vi "Abstract MVA Application (Template).vi"   [LabVIEW 2015]
uses:
  Framework/IModel/IModel/IModel.lvclass
  Framework/IViewable/IViewable/IViewable.lvclass
  Framework/IViewModel/IViewModel/IViewModel.lvclass
  Framework/Mediator/Mediator/Mediator.lvclass
  Framework/Mediator/MediatorBusMonitor/MediatorBusMonitor.lvclass
  <vilib>/ActorFramework/Message Enqueuer/Message Priority.ctl
  Framework/IViewable/IViewable/View Position Enum.ctl
  Framework/IMediator/IMediator/IMediator.lvclass/IMediator.ctl
  Framework/IViewModel/IViewModel/IViewModel.lvclass/IViewModel.ctl
  Framework/IViewManager/IViewManager Messages/Launch Nested Views Msg/Launch Nested Views Msg.lvclass/Launch Nested Views Msg.ctl
  Framework/IViewManager/IViewManager/IViewManager.lvclass/IViewManager.ctl
  Framework/IViewable/IViewable Messages/Open Front Panel Msg/Open Front Panel Msg.lvclass/Open Front Panel Msg.ctl
  <vilib>/ActorFramework/Message Enqueuer/Message Enqueuer.lvclass/Message Enqueuer.ctl
  Framework/IViewManager/IViewManager Messages/Launch Nested Views Msg/Pack Launch Nested Views Msg.vi
  Framework/IViewManager/IViewManager/Write Startup Launch Nested Views Msg.vi
  <vilib>/ActorFramework/Message Enqueuer/Enqueue.vi
  <vilib>/ActorFramework/Message Priority Queue/Priority Enqueue.vi
  Framework/IViewable/IApplicationStyle/IApplicationStyle.lvclass
  Framework/IViewManager/IViewManager Messages/Launch Nested Views Msg/Launch Nested Views Msg.lvclass
  Framework/IViewable/IViewable Messages/Open Front Panel Msg/Open Front Panel Msg.lvclass
  <vilib>/ActorFramework/Actor/Actor.lvclass
  Framework/IMediator/IMediator/IMediator.lvclass
  <vilib>/ActorFramework/Message Enqueuer/Message Enqueuer.lvclass
panel:
  # "This example launches a simple abstract MVA application.\nReplace IModel with your Root Model or dependency-injected Model hierarchy.\nReplace IViewable with your Viewable or nested hierarchy of Viewables and ViewManagers\nReplace IViewModel with your concrete ViewModel that requests Model activity driven by user inputs\nMediator is already concrete--only replace it if you write your own Mediator (highly unlikely)"
types:
  T1 = typedef "IViewable.lvlib/IViewable.lvclass/View Position Enum.ctl" = enum16{"Centered", "Maximized", "Minimized", "Custom", "Unchanged"}
  T2 = typedef "Actor Framework.lvlib/Message Enqueuer.lvclass/Message Priority.ctl" = enum16{"Low", "Normal", "High"}
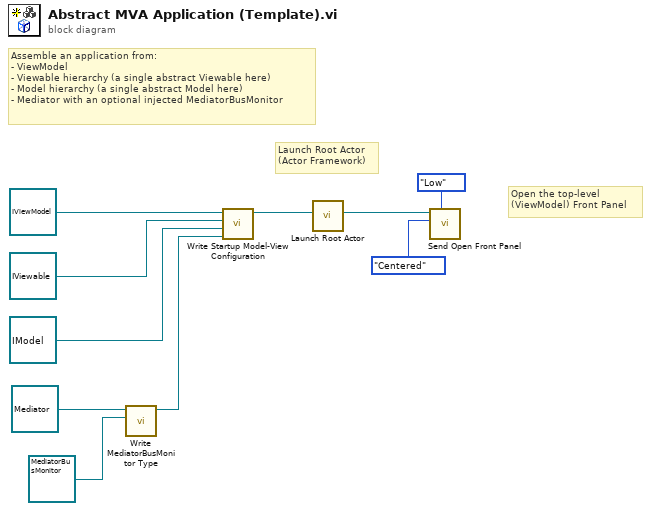
[diagram p0: block diagram]
diagram:
  # "Open the top-level\n(ViewModel) Front Panel"
  # "Launch Root Actor\n(Actor Framework)"
  # "Assemble an application from:\n- ViewModel\n- Viewable hierarchy (a single abstract Viewable here)\n- Model hierarchy (a single abstract Model here)\n- Mediator with an optional injected MediatorBusMonitor"
  n1 = call "Write MediatorBusMonitor Type.vi"("MediatorBusMonitor (Type)"=refnum<class "MediatorBusMonitor.lvclass"> refnum ("Mediator.lvlib:MediatorBusMonitor.lvclass"), "IMediator in"=refnum<class "Mediator.lvclass"> refnum ("Mediator.lvlib:Mediator.lvclass")) -> ("IMediator out"=w5:refnum<class "Mediator.lvclass">)  [unwired: 9 in]
  n2 = call "Write Startup Model-View Configuration.vi"("Mediator Type"=w5, "Model Type"=refnum<class "IModel.lvclass"> refnum ("IModel.lvlib:IModel.lvclass"), "Startup View Configuration"=refnum<class "IViewable.lvclass"> refnum ("IViewable.lvlib:IViewable.lvclass"), "IViewModel In"=refnum<class "IViewModel.lvclass"> refnum ("IViewModel.lvlib:IViewModel.lvclass")) -> ("IViewModel Out"=w4:refnum<class "IViewModel.lvclass">)  [unwired: 7 in]
  n3 = call <vilib>:"Launch Root Actor.vi"("Actor"=w4) -> ("Actor's Enqueuer"=w3:refnum<class "Message Enqueuer.lvclass">)  [unwired: 9 in, 1 out]
  n4 = call "Send Open Front Panel.vi"("Message Priority (Normal)"=Message_Priority."Low", "Position"=View_Position_Enum."Centered", "Message Enqueuer"=w3) -> ()  [unwired: 7 in, 2 out]
